vi "Untitled 2.vi"   [LabVIEW 2018, in "Copy of Actor.lvclass"]
uses:
  Copy of Actor.lvclass
types:
  T1 = cluster{"Some-Other-Name":refnum<event-registration>, "Event Registration Refnum":refnum<event-registration>}
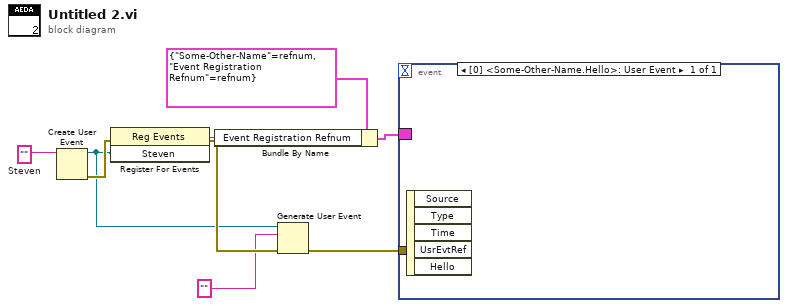
[diagram p0: block diagram]
diagram:
  w9 = ""  # Steven
  n1 = Create User Event(user event datatype=w9) -> (user event=w4:refnum<user-event>, error out=w8:errorcluster)  [unwired: 1 in]
  n2 = register-events(error in=w8, w4) -> (reference out=w2:refnum<event-registration>, error out=w7:errorcluster)  [unwired: 1 in]
  n3 = Bundle By Name(cluster=T1 {"Some-Other-Name"=refnum, "Event Registration Refnum"=refnum}, "Event Registration Refnum"=w2) -> (w1:T1)
  n4 = Generate User Event(user event=w4, event data cluster="" ("event data"), error in=w7) -> (error out=w6:errorcluster)  [unwired: 1 in, 1 out]
  n5 = event shown="[0] <Some-Other-Name.Hello>: User Event" {
    selector: w1 -> [_]
    dyn-events: _ -> [_]
    timeout: _ -> [_]
    tunnel: w6 -> [_]
    event User Event {
      n6 = event-data() -> ()  [unwired: 1 in, 5 out]
    }
  }
